vi "UploadAcquisitions.vi"(8 "error in (no error)":errorcluster, 10 "Acquisitions":T1, 11 "ByteGSAPIBase in":refnum<class "ByteQXAPIBase.lvclass">) -> (0 "error out":errorcluster, 3 "ByteGSAPIBase out":refnum<class "ByteQXAPIBase.lvclass">)   [LabVIEW 2019, in "ByteQXWebAPI.lvlib" / "ByteQXAPIBase.lvclass"]
uses:
  ByteQXAPIBase.lvclass
  acquisitions.ctl
  Private/module.ctl
  ByteQXAPIBase.lvclass/ByteQXAPIBase.ctl
  <vilib>/Bytelabs/ByteREST/ByteRESTClass/ByteRESTBase/RESTBase.lvclass
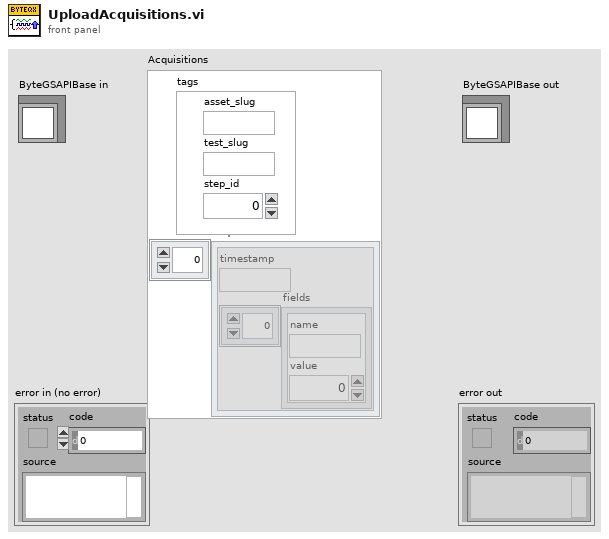
[diagram p1: front panel]
types:
  T1 = typedef "ByteQXWebAPI.lvlib/ByteQXAPIBase.lvclass/acquisitions.ctl" = cluster{"tags":cluster{"step_id":i32, "test_slug":string, "asset_slug":string}, "acquisitions":cluster{"timestamp":string, "fields":cluster{"name":string, "value":dbl}[]}[]}
  T2 = typedef "ByteQXWebAPI.lvlib/ByteQXAPIBase.lvclass/module.ctl" = enum16{"gs", "tms"}
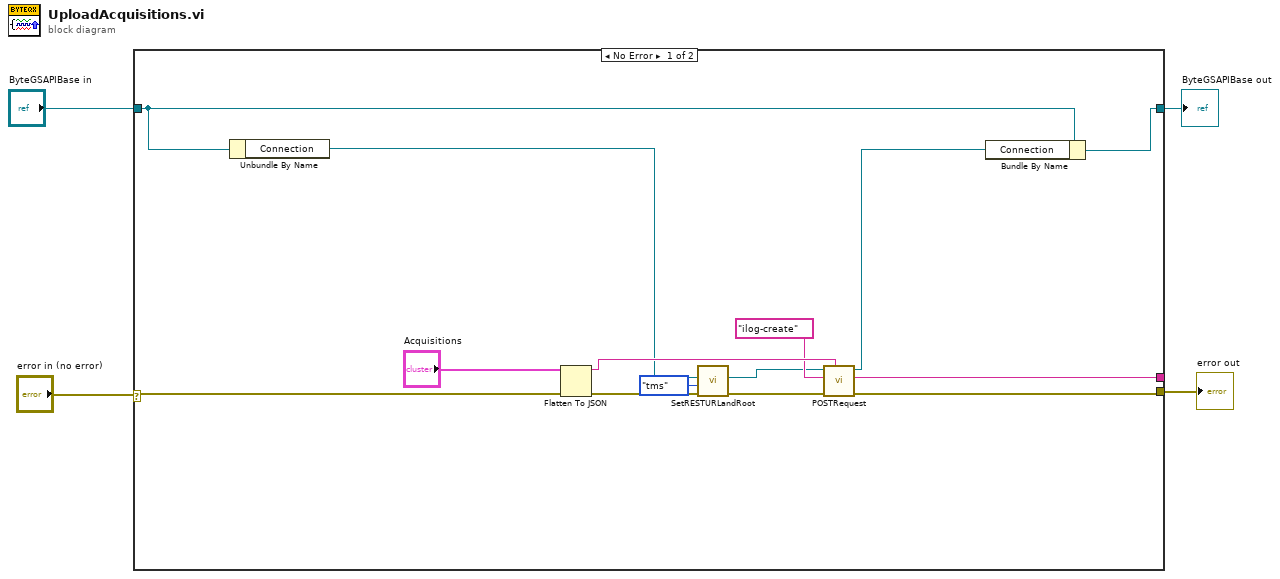
[diagram p0: block diagram]
diagram:
  n1 = case shown="No Error" "error in (no error)" {
    selector: "error in (no error)" -> [w14 w20]
    tunnel: [w12 w20] -> w3
    tunnel: [w17 w19] -> w1
    tunnel: "ByteGSAPIBase in" -> [w18 w19]
    tunnel: [w10 _] -> _
    frame No Error {
      n2 = Unbundle By Name(w18) -> ("Connection"=w7:refnum<class "RESTBase.lvclass">)
      n3 = Flatten To JSON(anything="Acquisitions", error in (no error)=w14) -> (JSON string=w16:string, 11:w9:errorcluster)  [unwired: 1 in]
      n4 = call "SetRESTURLandRoot.vi"("error in (no error)"=w9, "module"=module."tms", "ByteREST in"=w7) -> ("error out"=w8:errorcluster, "ByteREST out"=w6:refnum<class "RESTBase.lvclass">)  [unwired: 7 in]
      n5 = call-dynamic "POSTRequest.vi"("Body in"=w16, "error in (no error)"=w8, "Request"="ilog-create", "ByteRESTBase in"=w6) -> ("error out"=w12:errorcluster, "Body"=w10:string, "ByteRESTBase out"=w15:refnum<class "RESTBase.lvclass">)  [unwired: 4 in, 1 out]
      n6 = Bundle By Name(cluster=w18, "Connection"=w15) -> (w17:refnum<class "ByteQXAPIBase.lvclass">)
    }
    frame Error {
    }
  }
  "error out" <- w3
  "ByteGSAPIBase out" <- w1
